vi "Fluke 5080 AC DC Power Calibrator.vi"() -> ()   [LabVIEW 2012]
doc: "This example shows how to configure the calibrator to ac/dc power output mode."
uses:
  <instrlib>/Fluke 5080/Fluke 5080.lvlib
panel:
  in  "Phase Offset Type (0: Lead)":i32(ring) items=["Lead", "Lag"]
  in  "Power Factor (1.0)":dbl=0.8
  out "Power (watts)":dbl
  in  "Frequency (50.0 Hertz)":dbl=50.0
  in  "Phase (0.0 Degrees)":dbl=180.0
  in  "Current (1.0 A)":dbl=0.5
  in  "Primary Voltage (5.0)":dbl=1.0
  in  "Output Type (0: DC Volts)":i32(ring)=5 items=["DC Volts", "AC Volts", "DC Current", "AC Current", "DC Power", "AC Power", "Dual DC Volts", "Dual AC Volts", "Resistance"]
  in  "Low Terminal Tie Enabled (F: Disabled)":bool
  in  "Earth Ground Enabled (T: Enabled)":bool
  in  "Output Post Binding (0: AUX)":i32(ring) items=["AUX", "20A"]
  in  "Serial Configuration":T1={"Baud Rate"=9600, "Parity"=0, "Data Bits"=8, "Stop Bits"=10, "Flow Control"=0} {"Flow Control" items=["None", "XON/XOFF", "RTS/CTS", "XON/XOFF & RTS/CTS", "DTR/DSR", "XON/XOFF & DTR/DSR"]; "Stop Bits" items=["1.0"=10, "1.5"=15, "2.0"=20]; "Data Bits" items=["7"=7, "8"=8]; "Parity" items=["None", "Odd", "Even", "Mark", "Space"]; "Baud Rate" items=["300"=300, "600"=600, "1200"=1200, "2400"=2400, "4800"=4800, "9600"=9600, "19200"=19200]}
  in  "VISA resource name":refnum<visa-resource-name>
  # "(c) 2010 National Instruments.  ALL RIGHTS RESERVED."
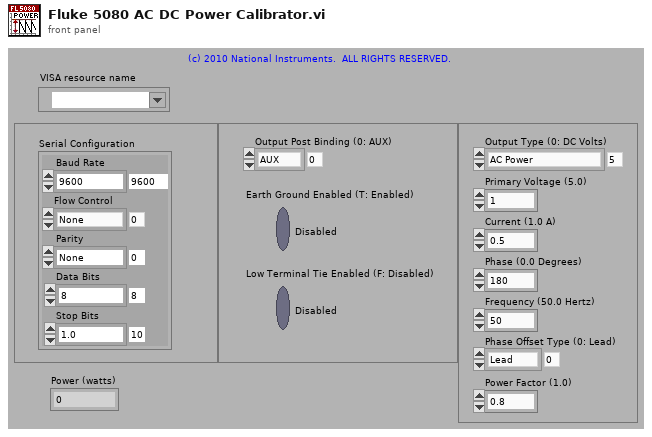
[diagram p1: front panel]
types:
  T1 = cluster{"Baud Rate":u32, "Parity":u16, "Data Bits":u16, "Stop Bits":u16, "Flow Control":u16}
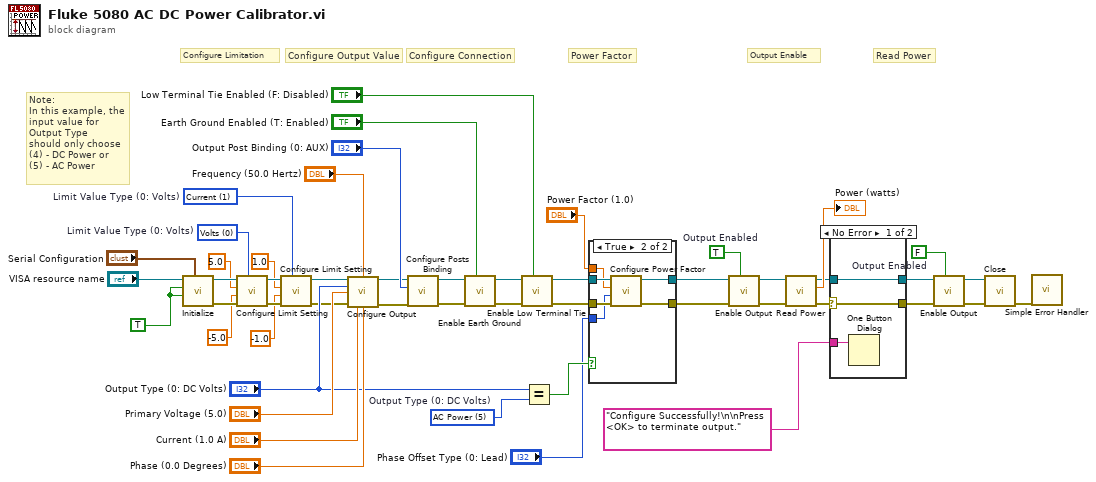
[diagram p0: block diagram]
diagram:
  w5 = 1 items=["Volts", "Current"]  # Limit Value Type (0: Volts)
  w10 = 0 items=["Volts", "Current"]  # Limit Value Type (0: Volts)
  w13 = FALSE  # Output Enabled
  w21 = TRUE  # Output Enabled
  w25 = 5 items=["DC Volts", "AC Volts", "DC Current", "AC Current", "DC Power", "AC Power", "Dual DC Volts", "Dual AC Volts", "Resistance"]  # Output Type (0: DC Volts)
  w49 = TRUE ("Reset (True)")
  # "Note:\nIn this example, the \ninput value for \nOutput Type\nshould only choose \n(4) - DC Power or \n(5) - AC Power"
  # "Read Power"
  # "Output Enable"
  # "Power Factor"
  # "Configure Connection"
  # "Configure Output Value"
  # "Configure Limitation"
  n1 = call <instrlib>:"Initialize.vi"("Serial Configuration"="Serial Configuration", "Reset (True)"=w49, "ID Query (True)"=w49, "VISA resource name"="VISA resource name") -> ("error out"=w40:errorcluster, "VISA resource name out"=w39:refnum<visa-resource-name>)  [unwired: 1 in, 5 out]
  n2 = call <instrlib>:"Configure Limit Setting.vi"("Limit Value Type (0: Volts)"=w10, "error in (no error)"=w40, "- Limit Value (-5)"=-5.0, "+ Limit Value (5)"=5.0, "VISA resource name"=w39) -> ("error out"=w6:errorcluster, "VISA resource name out"=w9:refnum<visa-resource-name>)  [unwired: 5 out]
  n3 = call <instrlib>:"Configure Limit Setting.vi"("Limit Value Type (0: Volts)"=w5, "error in (no error)"=w6, "- Limit Value (-5)"=-1.0, "+ Limit Value (5)"=1.0, "VISA resource name"=w9) -> ("error out"=w7:errorcluster, "VISA resource name out"=w8:refnum<visa-resource-name>)  [unwired: 5 out]
  n4 = call <instrlib>:"Configure Output.vi"("VISA resource name"=w8, "Frequency (50.0 Hertz)"="Frequency (50.0 Hertz)", "Output Type (0: DC Volts)"="Output Type (0: DC Volts)", "Primary Voltage (5.0)"="Primary Voltage (5.0)", "error in (no error)"=w7, "Current (1.0 A)"="Current (1.0 A)", "Phase (0.0 Degrees)"="Phase (0.0 Degrees)") -> ("VISA resource name out"=w32:refnum<visa-resource-name>, "error out"=w31:errorcluster)  [unwired: 3 in, 4 out]
  n5 = call <instrlib>:"Configure Posts Binding.vi"("error in (no error)"=w31, "Output Post Binding (0: AUX)"="Output Post Binding (0: AUX)", "VISA resource name"=w32) -> ("error out"=w46:errorcluster, "VISA resource name out"=w47:refnum<visa-resource-name>)  [unwired: 7 out]
  n6 = call <instrlib>:"Enable Earth Ground.vi"("Earth Ground Enabled (T: Enabled)"="Earth Ground Enabled (T: Enabled)", "error in (no error)"=w46, "VISA resource name"=w47) -> ("error out"=w44:errorcluster, "VISA resource name out"=w45:refnum<visa-resource-name>)  [unwired: 7 out]
  n7 = call <instrlib>:"Enable Low Terminal Tie.vi"("Low Terminal Tie Enabled (F: Disabled)"="Low Terminal Tie Enabled (F: Disabled)", "error in (no error)"=w44, "VISA resource name"=w45) -> ("error out"=w37:errorcluster, "VISA resource name out"=w38:refnum<visa-resource-name>)  [unwired: 7 out]
  n8 = Equal?(x="Output Type (0: DC Volts)", y=w25) -> (x = y?=w24:bool)
  n9 = case shown="True" w24 {
    tunnel: w38 -> [w52 w58]
    tunnel: w37 -> [w51 w57]
    tunnel: [w52 w56] -> w36
    tunnel: [w51 w55] -> w35
    tunnel: "Power Factor (1.0)" -> [_ w54]
    tunnel: "Phase Offset Type (0: Lead)" -> [_ w53]
    frame False {
    }
    frame True {
      n10 = call <instrlib>:"Configure Power Factor.vi"("error in (no error)"=w57, "Phase Offset Type (0: Lead)"=w53, "Power Factor (1.0)"=w54, "VISA resource name"=w58) -> ("error out"=w55:errorcluster, "VISA resource name out"=w56:refnum<visa-resource-name>)  [unwired: 6 out]
    }
  }
  n11 = call <instrlib>:"Enable Output.vi"("Output Enabled (T: Enable)"=w21, "error in (no error)"=w35, "VISA resource name"=w36) -> ("error out"=w33:errorcluster, "VISA resource name out"=w34:refnum<visa-resource-name>)  [unwired: 7 out]
  n12 = call <instrlib>:"Read Power.vi"("error in (no error)"=w33, "VISA resource name"=w34) -> ("error out"=w19:errorcluster, "Power (watts)"=→"Power (watts)":dbl, "VISA resource name out"=w18:refnum<visa-resource-name>)  [unwired: 7 out]
  n13 = case shown="No Error" w19 {
    selector: w19 -> [w60 w62]
    tunnel: "Configure Successfully!\n\nPress <OK> to terminate output." ("message") -> [w61 _]
    tunnel: [w60 w62] -> w15
    tunnel: [w59 w63] -> w17
    tunnel: w18 -> [w59 w63]
    frame No Error {
      n14 = One Button Dialog(message=w61) -> ()  [unwired: 2 out]
    }
    frame Error {
    }
  }
  n15 = call <instrlib>:"Enable Output.vi"("Output Enabled (T: Enable)"=w13, "error in (no error)"=w15, "VISA resource name"=w17) -> ("error out"=w14:errorcluster, "VISA resource name out"=w16:refnum<visa-resource-name>)  [unwired: 7 out]
  n16 = call <instrlib>:"Close.vi"("error in (no error)"=w14, "VISA resource name"=w16) -> ("error out"=w22:errorcluster)  [unwired: 9 out]
  n17 = call <vilib>:"Simple Error Handler.vi"("error in (no error)"=w22) -> ()  [unwired: 1 in, 8 out]
